vi "Practica 8.vi"() -> ()   [LabVIEW 2018]
uses:
  <vilib>/LabVIEW Interface for Arduino/Type Defs/Pin Mode.ctl
  <vilib>/LabVIEW Interface for Arduino/LabVIEW Interface for Arduino.lvlib
panel:
  out "Habilitada Salida":bool
  in  "stop":bool
  in  "Salida PIN 8":bool
  out "Reloj":bool
  in  "Tiempo":dbl
  # "Practica 8: Intermitente"
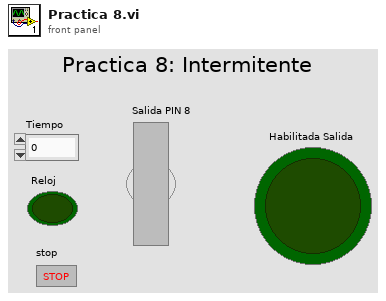
[diagram p1: front panel]
types:
  T1 = typedef "LabVIEW Interface for Arduino.lvlib/Pin Mode.ctl" = enum8{"Input", "Output"}
  T2 = typedef "LabVIEW Interface for Arduino.lvlib/Arduino Resource.ctl" = cluster{"VISA resource":refnum<visa-resource-name>, "Board Type":T3, "Connection Type":enum8{"USB / Serial"}, "Bytes Per Packet (15)":u8}
  T3 = typedef "LabVIEW Interface for Arduino.lvlib/Board Type.ctl" = enum16{"Uno", "Dimuelanove w/Atmega 328", "Mega 2560"}
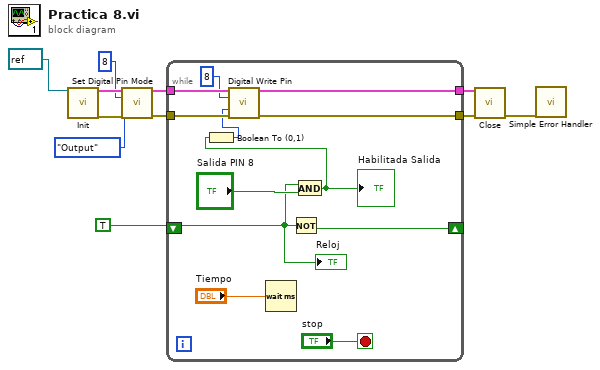
[diagram p0: block diagram]
diagram:
  n1 = call <vilib>:"Init.vi"("VISA resource"=refnum<visa-resource-name> refnum) -> ("Arduino Resource"=w11:T2, "error out"=w10:errorcluster)  [unwired: 17 in]
  n2 = call <vilib>:"Set Digital Pin Mode.vi"("Arduino Resource"=w11, "Digital I/O Pin"=u8 8, "Pin Mode (Input)"=Pin_Mode."Output", "error in"=w10) -> ("Arduino Resource"=w9:T2, "error out"=w8:errorcluster)  [unwired: 10 in]
  n3 = while {
    tunnel: w9 -> [w22]
    tunnel: w8 -> [w21]
    shift-right: [w15] -> _
    shift-left: TRUE -> [w16]
    tunnel: [w14] -> w4
    tunnel: [w13] -> w3
    stop <- "stop" stop-if-true
    n4 = Wait (ms)(milliseconds to wait="Tiempo") -> ()  [unwired: 1 out]
    n5 = Not(x=w16) -> (.not. x?=w15:bool)
    n6 = And(x=w16, y="Salida PIN 8") -> (x .and. y?=w12:bool)
    "Habilitada Salida" <- w12
    n7 = Boolean To (0,1)(Boolean=w12) -> (0, 1=w19:i16)
    n8 = call <vilib>:"Digital Write Pin.vi"("Arduino Resource"=w22, "Digital I/O Pin (0)"=u8 8, "Value (0)"=w19, "error in"=w21) -> ("Arduino Resource"=w14:T2, "error out"=w13:errorcluster)  [unwired: 10 in]
    "Reloj" <- w16
  }
  n9 = call <vilib>:"Close.vi"("Arduino Resource"=w4, "error in"=w3) -> ("error out"=w2:errorcluster)  [unwired: 13 in]
  n10 = call <vilib>:"Simple Error Handler.vi"("error in (no error)"=w2) -> ()  [unwired: 4 in, 5 out]
